vi "PostFireSeq.vi"() -> ()   [LabVIEW 2016]
panel:
  in  "String":string
  out "Purge Valves":bool[](array[boolean])
  out "Main Valves":bool[](array[boolean])
  in  "Ox N2 Flow":bool
  in  "Fuel N2 Flow":bool
  in  "Oxygen Purge":bool
  in  "Fuel Purge":bool
  in  "ABORT":bool
  in  "F Purge":bool
  in  "O Purge":bool
  out "Ox Purged":bool
  out "Fuel Purged":bool
  # "Fuel:"
  # "Purge"
  # "N2 Flow"
  # "Oxidizer"
  # "Purge"
  # "N2 Flow"
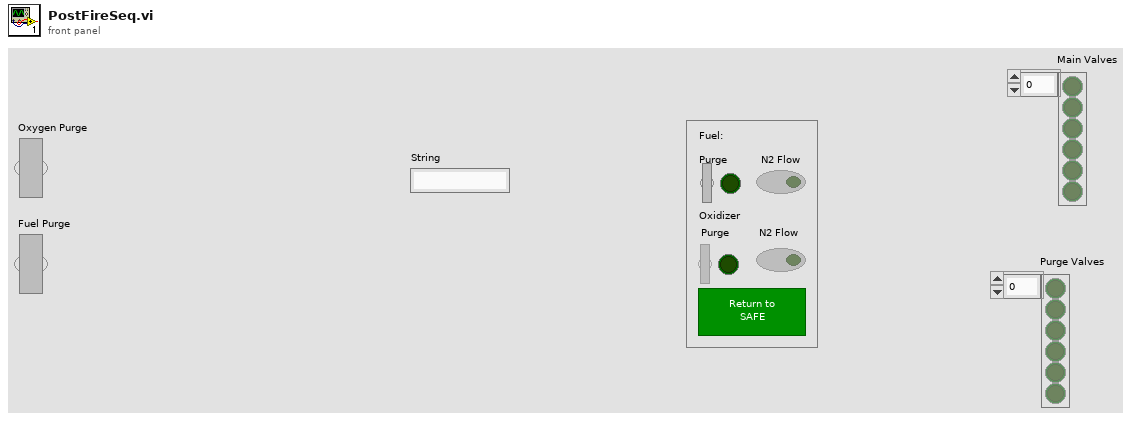
[diagram p1: front panel]
types:
  T1 = enum8{"Enabled", "Disabled", "Disabled and Grayed Out"}
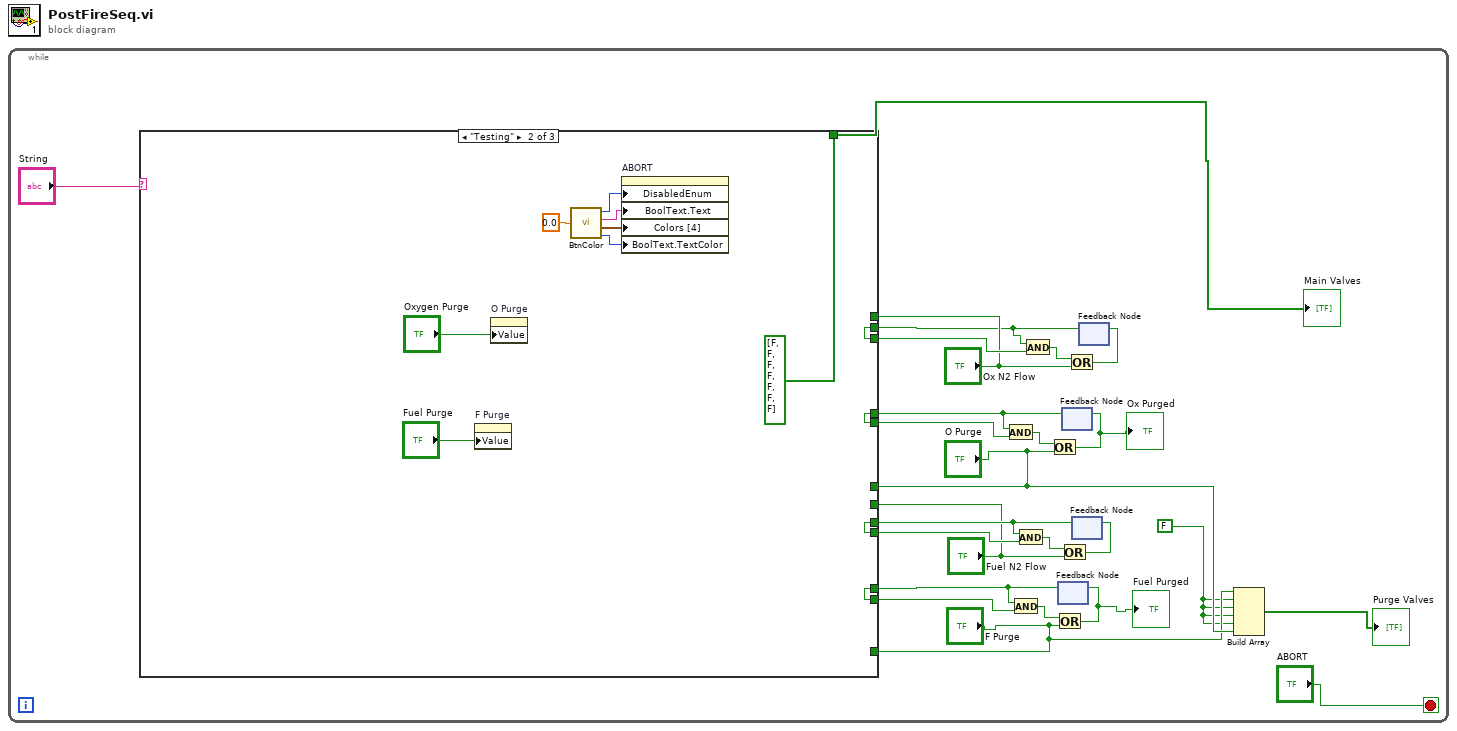
[diagram p0: block diagram]
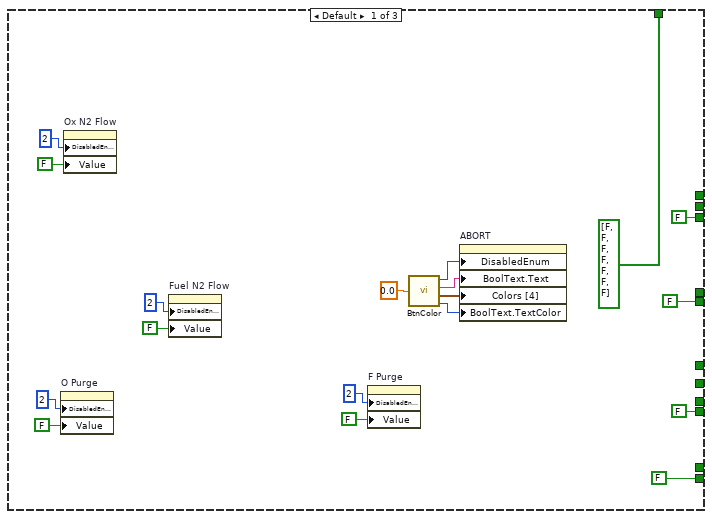
[diagram p2: hidden frame]
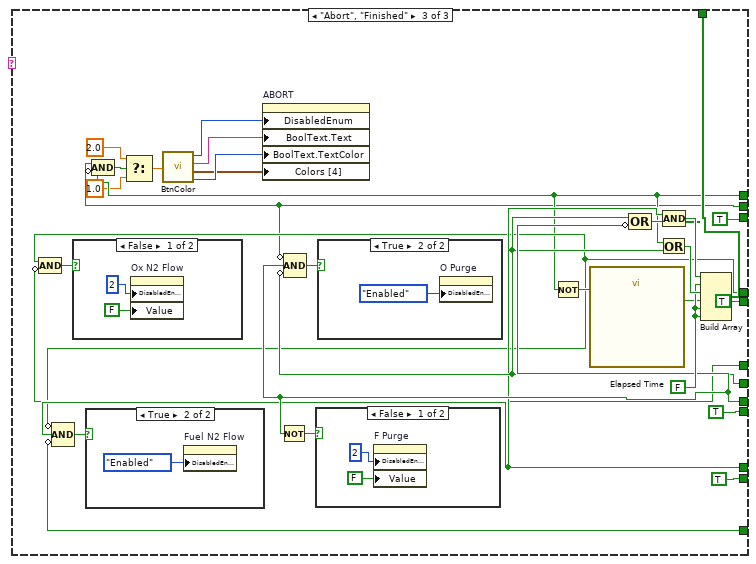
[diagram p3: hidden frame]
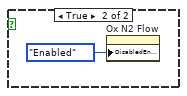
[diagram p4: hidden frame]
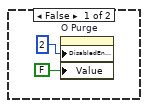
[diagram p5: hidden frame]
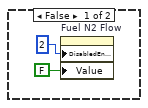
[diagram p6: hidden frame]
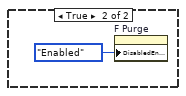
[diagram p7: hidden frame]
diagram:
  n1 = while {
    stop <- "ABORT" stop-if-true
    w1 = FALSE
    n2 = feedback #1() -> (w10:bool)  [unwired: 1 in]
    n3 = feedback #2() -> (w21:bool)  [unwired: 1 in]
    n4 = feedback #3() -> (w11:bool)  [unwired: 1 in]
    n5 = feedback #4() -> (w9:bool)  [unwired: 1 in]
    n6 = case shown="\"Testing\"" "String" {
      tunnel: [FALSE w55 TRUE] -> w23
      tunnel: [FALSE w54 TRUE] -> w22
      tunnel: [bool[] [FALSE, FALSE, FALSE, FALSE, FALSE, FALSE, FALSE] bool[] [FALSE, FALSE, FALSE, FALSE, FALSE, FALSE, FALSE] w84] -> w4
      tunnel: w21 -> [_ w55 w68]
      tunnel: w10 -> [_ w54 w70]
      tunnel: w9 -> [_ w52 w66]
      tunnel: [FALSE w52 TRUE] -> w16
      tunnel: w11 -> [_ w51 w72]
      tunnel: [FALSE w51 TRUE] -> w13
      tunnel: "Fuel N2 Flow" -> [_ _ w71]
      tunnel: "Ox N2 Flow" -> [_ _ w67]
      tunnel: "O Purge" -> [_ _ w69]
      tunnel: "F Purge" -> [_ _ w73]
      frame Default {
        n7 = property on="O Purge" class="Bool (strict)"("DisabledEnum"=2, "Value"=FALSE ("F Purge")) -> ()  [unwired: 2 in, 2 out]
        n8 = property on="Ox N2 Flow" class="Bool (strict)"("DisabledEnum"=2, "Value"=FALSE ("F Purge")) -> ()  [unwired: 2 in, 2 out]
        n9 = property on="Fuel N2 Flow" class="Bool (strict)"("DisabledEnum"=2, "Value"=FALSE ("F Purge")) -> ()  [unwired: 2 in, 2 out]
        n10 = property on="F Purge" class="Bool (strict)"("DisabledEnum"=2, "Value"=FALSE ("F Purge")) -> ()  [unwired: 2 in, 2 out]
        n11 = call "BtnColor.vi"("Selector"=0.0) -> ("Text Color"=w38:i32, "Colors"=w37:cluster{u32, u32}[], "Text"=w39:string, "Disabled"=w40:i32)  [unwired: 4 in]
        n12 = property on="ABORT" class="Bool"("DisabledEnum"=w40, "BoolText.Text"=w39, "Colors [4]"=w37, "BoolText.TextColor"=w38) -> ()  [unwired: 2 in, 2 out]
      }
      frame "Testing" {
        n13 = property on="F Purge" class="Bool (strict)"("Value"="Fuel Purge") -> ()  [unwired: 2 in, 2 out]
        n14 = property on="O Purge" class="Bool (strict)"("Value"="Oxygen Purge") -> ()  [unwired: 2 in, 2 out]
        n15 = call "BtnColor.vi"("Selector"=0.0) -> ("Text Color"=w46:i32, "Colors"=w45:cluster{u32, u32}[], "Text"=w47:string, "Disabled"=w48:i32)  [unwired: 4 in]
        n16 = property on="ABORT" class="Bool"("DisabledEnum"=w48, "BoolText.Text"=w47, "Colors [4]"=w45, "BoolText.TextColor"=w46) -> ()  [unwired: 2 in, 2 out]
      }
      frame "Abort", "Finished" {
        w78 = FALSE
        n17 = Compound Arithmetic op=AND(w68, invert w69) -> (w56:bool)
        n18 = Compound Arithmetic op=AND(invert w68, w70, invert w73) -> (w74:bool)
        n19 = case shown="False" w56 {
          frame False {
            n20 = property on="Ox N2 Flow" class="Bool (strict)"("DisabledEnum"=2, "Value"=FALSE ("F Purge")) -> ()  [unwired: 2 in, 2 out]
          }
          frame True {
            n21 = property on="Ox N2 Flow" class="Bool (strict)"("DisabledEnum"=T1."Enabled" ("Disabled")) -> ()  [unwired: 2 in, 2 out]
          }
        }
        n22 = case shown="True" w74 {
          frame False {
            n23 = property on="Fuel N2 Flow" class="Bool (strict)"("DisabledEnum"=2, "Value"=FALSE ("F Purge")) -> ()  [unwired: 2 in, 2 out]
          }
          frame True {
            n24 = property on="Fuel N2 Flow" class="Bool (strict)"("DisabledEnum"=T1."Enabled" ("Disabled")) -> ()  [unwired: 2 in, 2 out]
          }
        }
        n25 = Compound Arithmetic op=AND(w66, invert w67) -> (w60:bool)
        n26 = Select(t=2.0, s=w60, f=1.0) -> (s? t:f=w61:dbl)
        n27 = call "BtnColor.vi"("Selector"=w61) -> ("Text Color"=w65:i32, "Colors"=w64:cluster{u32, u32}[], "Text"=w63:string, "Disabled"=w62:i32)  [unwired: 4 in]
        n28 = property on="ABORT" class="Bool"("DisabledEnum"=w62, "BoolText.Text"=w63, "BoolText.TextColor"=w65, "Colors [4]"=w64) -> ()  [unwired: 2 in, 2 out]
        n29 = Not(x=w72) -> (.not. x?=w75:bool)
        n30 = Compound Arithmetic op=AND(invert w66, w72, invert w71) -> (w57:bool)
        n31 = case shown="False" w75 {
          frame False {
            n32 = property on="F Purge" class="Bool (strict)"("DisabledEnum"=2, "Value"=FALSE ("F Purge")) -> ()  [unwired: 2 in, 2 out]
          }
          frame True {
            n33 = property on="F Purge" class="Bool (strict)"("DisabledEnum"=T1."Enabled" ("Disabled")) -> ()  [unwired: 2 in, 2 out]
          }
        }
        n34 = case shown="True" w57 {
          frame False {
            n35 = property on="O Purge" class="Bool (strict)"("DisabledEnum"=2, "Value"=FALSE ("F Purge")) -> ()  [unwired: 2 in, 2 out]
          }
          frame True {
            n36 = property on="O Purge" class="Bool (strict)"("DisabledEnum"=T1."Enabled" ("Disabled")) -> ()  [unwired: 2 in, 2 out]
          }
        }
        n37 = Not(x=w67) -> (.not. x?=w77:bool)
        n38 = call "Elapsed Time"("Reset"=w77) -> ("Time has Elapsed"=w76:bool)  [unwired: 11 in, 7 out]
        n39 = Compound Arithmetic op=OR(w71, invert w72) -> (w80:bool)
        n40 = Or(x=w67, y=w71) -> (x .or. y?=w79:bool)
        n41 = Compound Arithmetic op=AND(w70, w80) -> (w81:bool)
        n42 = Build Array(w81, w78, w79, w76, w78, w78) -> (w84:bool[])
      }
    }
    "Main Valves" <- w4
    n43 = And(x=w21, y=w23) -> (x .and. y?=w25:bool)
    n44 = And(x=w10, y=w22) -> (x .and. y?=w24:bool)
    n45 = And(x=w11, y=w13) -> (x .and. y?=w15:bool)
    n46 = And(x=w9, y=w16) -> (x .and. y?=w18:bool)
    n47 = Or(x=w25, y="O Purge") -> (x .or. y?=w19:bool)
    "Ox Purged" <- w19
    n48 = Or(x=w24, y="F Purge") -> (x .or. y?=w20:bool)
    "Fuel Purged" <- w20
    n49 = feedback-in #1(w20) -> ()
    n50 = Or(x=w15, y="Fuel N2 Flow") -> (x .or. y?=w14:bool)
    n51 = feedback-in #2(w19) -> ()
    n52 = Or(x=w18, y="Ox N2 Flow") -> (x .or. y?=w17:bool)
    n53 = feedback-in #3(w14) -> ()
    n54 = feedback-in #4(w17) -> ()
    n55 = Build Array("F Purge", w1, w1, w1, w1, "O Purge") -> (→"Purge Valves":bool[])
  }
